vi "Configure Active Step Parameters.vi"(0 "VISA resource name":refnum<visa-resource-name>, 5 "Step (1)":i32=1 min=1 max=9 step=1, 7 "Step Cycle (1)":i32=1 min=0 max=9999 step=1, 9 "Enable Step Connection (F:Disable)":bool, 11 "error in (no error)":errorcluster) -> (4 "VISA resource name out":refnum<visa-resource-name>, 15 "error out":errorcluster)   [LabVIEW 2016, in "APT 300XAC Series.lvlib"]
doc: "Configures <B>active step, step cycle and Step connect mode</B> in the current Memory location (Use \"Configure Memory.vi\" to select the desired memory)\n\nSelect the active step in the step control available in this VI so that the desired step is made active for configuration\n\nNote : This VI should be used only in Program mode."
uses:
  APT 300XAC Series.lvlib
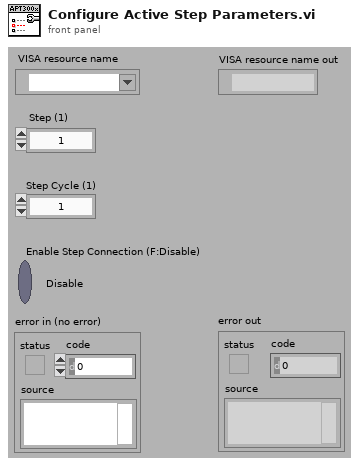
[diagram p1: front panel]
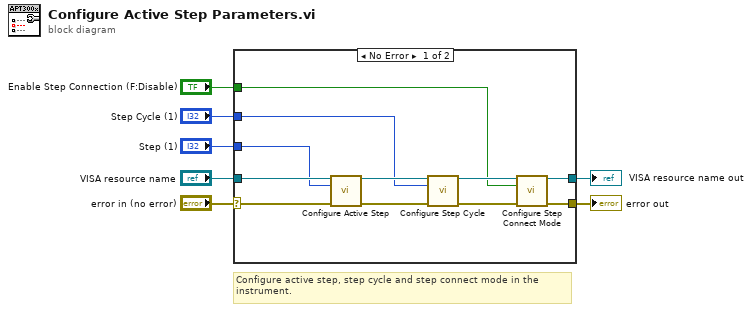
[diagram p0: block diagram]
diagram:
  # "Configure active step, step cycle and step connect mode in the \ninstrument."
  n1 = case shown="No Error" "error in (no error)" {
    selector: "error in (no error)" -> [w11 w19]
    tunnel: [w18 w19] -> w7
    tunnel: [w17 w20] -> w6
    tunnel: "VISA resource name" -> [w12 w20]
    tunnel: "Step (1)" -> [w10 _]
    tunnel: "Step Cycle (1)" -> [w9 _]
    tunnel: "Enable Step Connection (F:Disable)" -> [w8 _]
    frame No Error {
      n2 = call "Configure Active Step.vi"("VISA resource name"=w12, "Step (1)"=w10, "error in (no error)"=w11) -> ("VISA resource name out"=w13:refnum<visa-resource-name>, "error out"=w14:errorcluster)  [unwired: 11 in]
      n3 = call "Configure Step Cycle.vi"("VISA resource name"=w13, "Step Cycle (1)"=w9, "error in (no error)"=w14) -> ("VISA resource name out"=w15:refnum<visa-resource-name>, "error out"=w16:errorcluster)  [unwired: 11 in]
      n4 = call "Configure Step Connect Mode.vi"("VISA resource name"=w15, "Enable Step Connection (F:Disable)"=w8, "error in (no error)"=w16) -> ("VISA resource name out"=w17:refnum<visa-resource-name>, "error out"=w18:errorcluster)  [unwired: 11 in]
    }
    frame Error {
    }
  }
  "error out" <- w7
  "VISA resource name out" <- w6
